vi "Texture_GetTextures.vi"(11 "Texture Path":path) -> (2 "Texture Bank 1":u8[](array[numeric]), 3 "Texture Bank 0":u8[](array[numeric]))   [LabVIEW 2020]
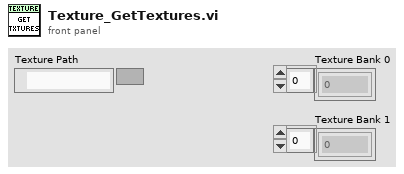
[diagram p1: front panel]
types:
  T1 = typedef "imagedata.ctl" = cluster{"image type":i32, "image depth":i32, "image":u8[], "mask":u8[], "colors":u32[], "Rectangle":cluster{"left":i16, "top":i16, "right":i16, "bottom":i16}}
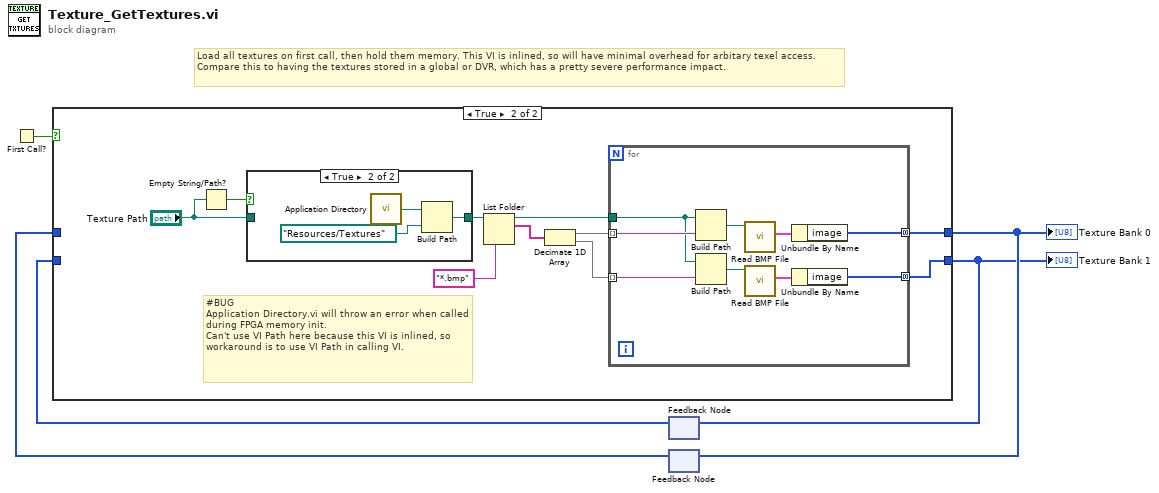
[diagram p0: block diagram]
diagram:
  # "Load all textures on first call, then hold them memory. This VI is inlined, so will have minimal overhead for arbitary texel access. Compare this to having the textures stored in a global or DVR, which has a pretty severe performance impact."
  n1 = First Call?() -> (First Call?: T/F=w5:bool)
  n2 = feedback #1() -> (w1:u8[])  [unwired: 1 in]
  n3 = feedback #2() -> (w4:u8[])  [unwired: 1 in]
  n4 = case shown="True" w5 {
    tunnel: [w7 w17] -> w3
    tunnel: w4 -> [w7 _]
    tunnel: [w6 w10] -> w2
    tunnel: w1 -> [w6 _]
    frame False {
    }
    frame True {
      # "#BUG\nApplication Directory.vi will throw an error when called during FPGA memory init.\nCan't use VI Path here because this VI is inlined, so workaround is to use VI Path in calling VI."
      n5 = Empty String/Path?(string/path="Texture Path") -> (empty?=w9:bool)
      n6 = case shown="True" w9 {
        tunnel: [w18 w20] -> w13
        tunnel: "Texture Path" -> [w18 _]
        frame False {
        }
        frame True {
          n7 = call <vilib>:"Application Directory.vi"() -> ("Application Directory"=w19:path)
          n8 = Build Path(base path=w19, name or relative path=path "Resources/Textures") -> (appended path=w20:path)
        }
      }
      n9 = List Folder(path=w13, pattern="*.bmp") -> (path out=w15:path, filenames=w14:string[])  [unwired: 2 in, 2 out]
      n10 = Decimate 1D Array(w14) -> (w12:string[], w11:string[])
      n11 = for {
        tunnel: w12 -> [w30] mode=indexing
        tunnel: [w29] -> w17 mode=concatenating
        tunnel: w15 -> [w27]
        tunnel: w11 -> [w28] mode=indexing
        tunnel: [w26] -> w10 mode=concatenating
        n12 = Build Path(base path=w27, name or relative path=w30) -> (appended path=w25:path)
        n13 = Build Path(base path=w27, name or relative path=w28) -> (appended path=w22:path)
        n14 = call <vilib>:"Read BMP File.vi"("path to BMP file"=w25) -> ("image data"=w24:T1)  [unwired: 8 in, 2 out]
        n15 = call <vilib>:"Read BMP File.vi"("path to BMP file"=w22) -> ("image data"=w23:T1)  [unwired: 8 in, 2 out]
        n16 = Unbundle By Name(w24) -> ("image"=w29:u8[])
        n17 = Unbundle By Name(w23) -> ("image"=w26:u8[])
      }
    }
  }
  "Texture Bank 0" <- w3
  "Texture Bank 1" <- w2
  n18 = feedback-in #1(w2) -> ()
  n19 = feedback-in #2(w3) -> ()
